vi "SWERVE DRIVE AUTO.vi"(8 "error in (no error)":errorcluster, 11 "auto pgm array":T4[](array[typedef])=[{"auto drive command"={"TRANSLATE"={"drive\ndistance (ft)"=10.0, "steer\nbearing (deg)"=0.0, "max strafe\nvelocity (ft/s)"=10.0, "max strafe\naccel (ft/s^2)"=58.7}, "ROTATE"={"rotate to\nbearing (deg)"=0.0, "max rotate\nvelocity (deg/s)"=0.0, "max rotate\naccel (ft/s^2)"=25.0}}, "sub-systems"={"start INTAKE"=FALSE, "extend FLAP"=FALSE, "SHOOT"=FALSE, "retract FLAP"=FALSE, "TARGET SPEAKER"=FALSE, "TARGET AMP"=FALSE, "TARGET OFF"=FALSE, "DANCE"=FALSE}}, {"auto drive command"={"TRANSLATE"={"drive\ndistance (ft)"=5.0, "steer\nbearing (deg)"=180.0, "max strafe\nvelocity (ft/s)"=5.0, "max strafe\naccel (ft/s^2)"=58.7}, "ROTATE"={"rotate to\nbearing (deg)"=0.0, "max rotate\nvelocity (deg/s)"=180.0, "max rotate\naccel (ft/s^2)"=25.0}}, "sub-systems"={"start INTAKE"=FALSE, "extend FLAP"=FALSE, "SHOOT"=FALSE, "retract FLAP"=FALSE, "TARGET SPEAKER"=FALSE, "TARGET AMP"=FALSE, "TARGET OFF"=FALSE, "DANCE"=FALSE}}] {"auto drive command"."ROTATE"."max rotate\naccel (ft/s^2)" min=0.0 max=200.0 step=0.1 format="%_3f"; "auto drive command"."ROTATE"."max rotate\nvelocity (deg/s)" min=0.0 step=0.001; "auto drive command"."TRANSLATE"."max strafe\naccel (ft/s^2)" min=0.0 max=200.0 step=0.1 format="%_3f"; "auto drive command"."TRANSLATE"."max strafe\nvelocity (ft/s)" min=0.0 max=20.0 step=0.001 format="%_5f"}) -> (0 "error out":errorcluster)   [LabVIEW 2023]
uses:
  ctrl defs/ctrl AUTONOMOUS step control.ctl
  ctrl defs/ctrl AUTONOMOUS drive step control.ctl
  ctrl defs/ctrl AUTONOMOUS systems step control.ctl
  ctrl defs/ctrl AUTO STATES.ctl
  <vilib>/Rock Robotics/WPI/ThirdParty/REV Robotics/REVLib/Typedef/Spark MAX Smart Motion Parameters.ctl
  <vilib>/Rock Robotics/WPI/ThirdParty/REV Robotics/REVLib/Typedef/Spark MAX Control Type.ctl
  Global INIT.vi
  Global odometry.vi
  <vilib>/Rock Robotics/WPI/ThirdParty/Phoenix-LabVIEW/CANCoder/Get/CTRE_Phoenix_CANcoder_GetSensorData.vi
  Global stack names.vi
  <vilib>/Rock Robotics/Network Tables/NT Read Boolean.vi
panel:
  out "Sensor Velocity":dbl[](array[numeric])
  in  "Smart Motion Parameters":T1
  in  "PID Constants":T2={"P Gain"=0.0, "I Gain"=0.0, "D Gain"=0.0, "F Gain"=0.0, "I Zone"=0.0, "Min Output"=-1.0, "Max Output"=1.0} {"Max Output" min=0.0 max=1.0 step=0.01; "Min Output" min=-1.0 max=0.0 step=0.01}
  in  "loop exit":bool
  in  "STATE":T3
  out "wheel\npos (rev)":dbl[](array[numeric])
  out "@ target":bool[](array[boolean])
  out "pos\ntarget (rev)":dbl[](array[numeric])
  out "rev tol\nto target":dbl
  out "distance (ft)\nto wheel revs":dbl
  out "vel to wheel\nspeed\n(rpm per ft/s)":dbl
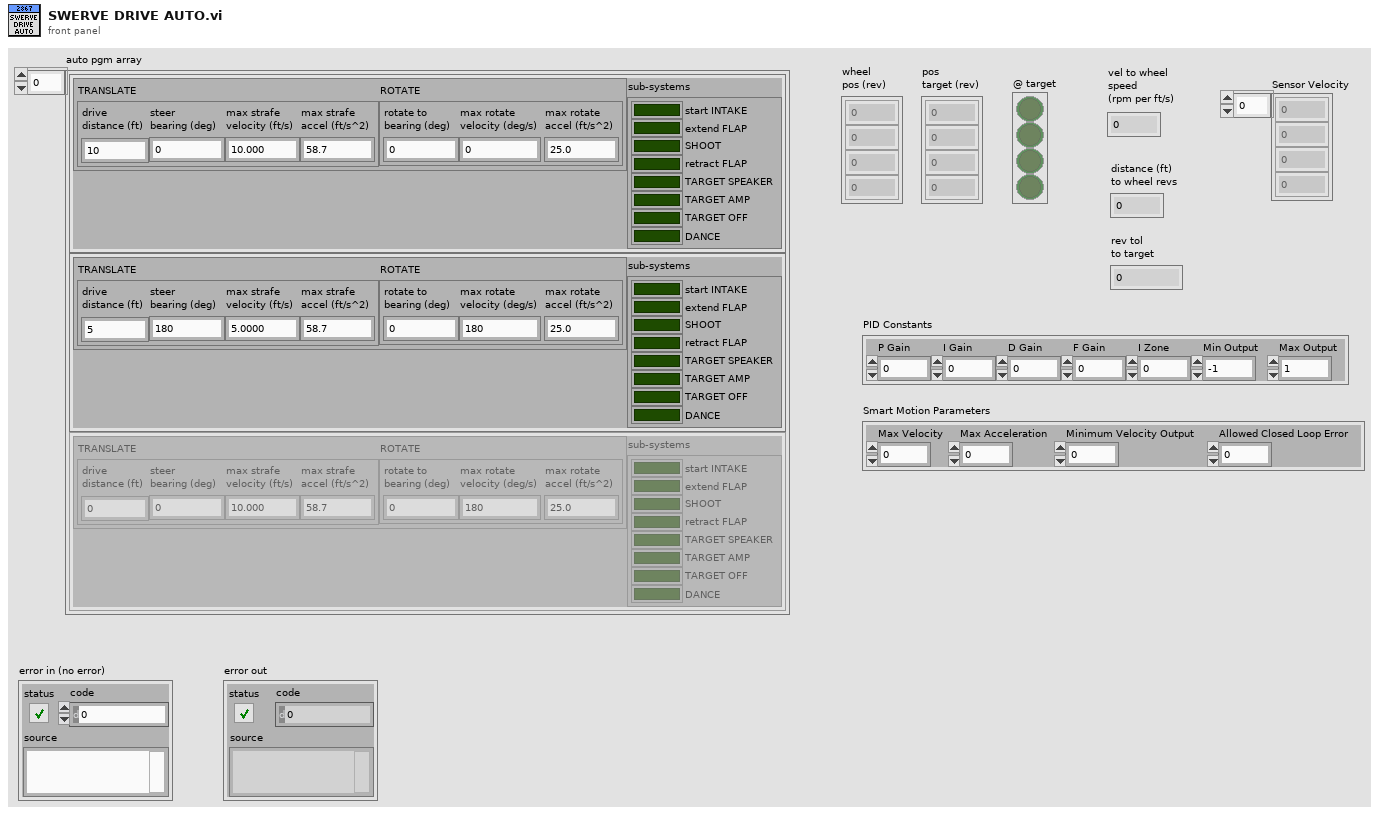
[diagram p1: front panel]
types:
  T1 = typedef "Spark MAX Smart Motion Parameters.ctl" = cluster{"Max Velocity":dbl, "Max Acceleration":dbl, "Minimum Velocity Output":dbl, "Allowed Closed Loop Error":dbl}
  T2 = cluster{"P Gain":dbl, "I Gain":dbl, "D Gain":dbl, "F Gain":dbl, "I Zone":dbl, "Min Output":dbl, "Max Output":dbl}
  T3 = typedef "ctrl AUTO STATES.ctl" = enum16{"TRANSLATE", "ROTATE", "TARGET", "INTAKE", "SHOOT", "DANCE", "WAIT for INTAKE", "WAIT for SHOOTER", "END", "SUB-SYSTEMS"}
  T4 = typedef "ctrl AUTONOMOUS step control.ctl" = cluster{"auto drive command":T5, "sub-systems":T6}
  T5 = typedef "ctrl AUTONOMOUS drive step control.ctl" = cluster{"TRANSLATE":cluster{"drive\ndistance (ft)":dbl, "steer\nbearing (deg)":dbl, "max strafe\nvelocity (ft/s)":dbl, "max strafe\naccel (ft/s^2)":dbl}, "ROTATE":cluster{"rotate to\nbearing (deg)":dbl, "max rotate\nvelocity (deg/s)":dbl, "max rotate\naccel (ft/s^2)":dbl}}
  T6 = typedef "ctrl AUTONOMOUS systems step control.ctl" = cluster{"start INTAKE":bool, "extend FLAP":bool, "SHOOT":bool, "retract FLAP":bool, "TARGET SPEAKER":bool, "TARGET AMP":bool, "TARGET OFF":bool, "DANCE":bool}
  T7 = typedef "ctrl swerve motor.ctl" = cluster{"description":string, "MOTOR SELECT":T8, "Installed?":bool, "CAN ID":u8, "refnum name":string, "Invert":bool, "Idle Mode":T9, "Current limiting":T10, "MOTOR PIDF coefficients":T11, "gear ratio":dbl}
  T8 = typedef "ctrl MOTOR SELECT.ctl" = i16
  T9 = typedef "Spark MAX Idle Mode.ctl" = enum16{"Coast", "Brake"}
  T10 = typedef "ctrl Spark MAX current limiting.ctl" = cluster{"Linearized":bool, "Free Speed (A)":dbl, "Primay (A)":dbl, "Limit RPM (0)":u32}
  T11 = typedef "ctrl motor PIDF coefficients.ctl" = cluster{"PIDF":cluster{"P Gain":dbl, "I Gain":dbl, "D Gain":dbl, "F Gain":dbl, "I Zone":dbl, "Min Output":dbl, "Max Output":dbl}, "Smart Motion":T1}
  T12 = typedef "ctrl swerve module.ctl" = cluster{"descr":string, "V":dbl, "POS":dbl, "target":dbl, "ABS":dbl, "from pivot to module":cluster{"R":dbl, "theta (deg)":dbl, "theta spin (deg)":dbl, "theta park (deg)":dbl}, "coord wrt geom CTR":cluster{"X":dbl, "Y":dbl}, "corner wt (lbm)":dbl}
  T13 = typedef "WPI_MotorControlDeviceRef.ctl" = cluster{"DeviceStatus":errorcluster, "Type":T14, "PWM":cluster{"PWM Channel":T15, "DeadBand":T16}, "CAN":cluster{"Device Number":u8, "SetOutput VI Ref":variant, "GetOutput VI Ref":variant, "Enable VI Ref":variant, "Disable VI Ref":variant, "Data":variant}, "Invert":bool, "DIO PWM":cluster{"PWM \"Enable\" Channel":T15, "DIOChannel":T17, "PWM Rate":dbl}}
  T14 = typedef "WPI_MotorControlType.ctl" = enum16{"PWM", "CAN", "DIO PWM"}
  T15 = typedef "FPGA_DIOPWMChannel.ctl" = enum8{"PWM 0", "PWM 1", "PWM 2", "PWM 3", "PWM 4", "PWM 5", "PWM 6", "PWM 7", "PWM 8", "PWM 9", "PWM MXP 0", "PWM MXP 1", "PWM MXP 2", "PWM MXP 3", "PWM MXP 4", "PWM MXP 5", "PWM MXP 6", "PWM MXP 7", "PWM MXP 8", "PWM MXP 9", "Invalid"}
  T16 = typedef "WPI_PWMDeadband.ctl" = cluster{"Name":string, "maxPositivePwm":i32, "minPositivePwm":i32, "centerPwm":i32, "maxNegativePwm":i32, "minNegativePwm":i32, "angularRange":u16}
  T17 = typedef "FPGA_DIOChannel.ctl" = enum8{"DIO 0", "DIO 1", "DIO 2", "DIO 3", "DIO 4", "DIO 5", "DIO 6", "DIO 7", "DIO 8", "DIO 9", "DIO MXP 0", "DIO MXP 1", "DIO MXP 2", "DIO MXP 3", "DIO MXP 4", "DIO MXP 5", "DIO MXP 6", "DIO MXP 7", "DIO MXP 8", "DIO MXP 9", "DIO MXP 10", "DIO MXP 11", "DIO MXP 12", "DIO MXP 13", "DIO MXP 14", "DIO MXP 15", "SPI Port CS1", "SPI Port CS2", "SPI Port CS3", "SPI Port MISO", "SPI Port MOSI", "Invalid"}
  T18 = typedef "CTRE_Phoenix_CANcoder_DeviceRef.ctl" = cluster{"DeviceStatus":errorcluster, "Device Number":u8, "Handle":u64, "UsageFrame":u32, "Library Path":path}
  T19 = cluster{"Driver":T13, "Steer":T13, "Encoder":T18}[]
  T20 = typedef "Spark MAX Control Type.ctl" = enum16{"Percent VBus", "Voltage", "Velocity", "Position", "Smart Motion", "Current", "Smart Velocity"}
  T21 = typedef "ctrl stack - INTAKE SHOOTER.ctl" = cluster{"INTAKE STATE":string, "RUN INTAKE?":string, "RUN REVERSE?":string, "NOTE LOADED?":string, "SHOOTER STATE":string, "SHOOTER FIRE?":string, "SHOOT AMP?":string, "EXTEND FLAP?":string, "LOOKING for NOTE":string}
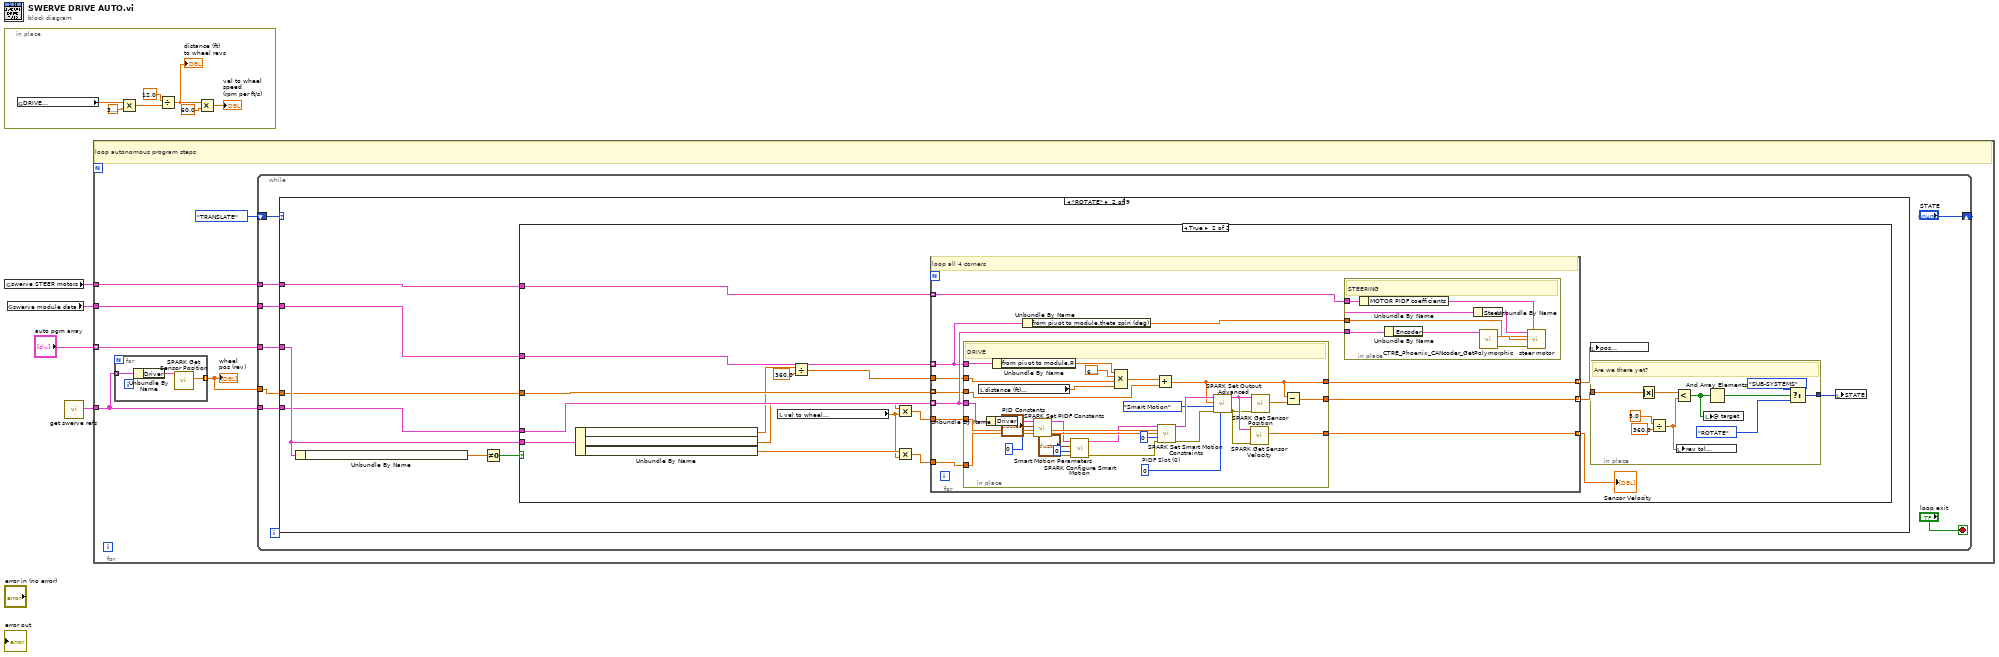
[diagram p0: block diagram]
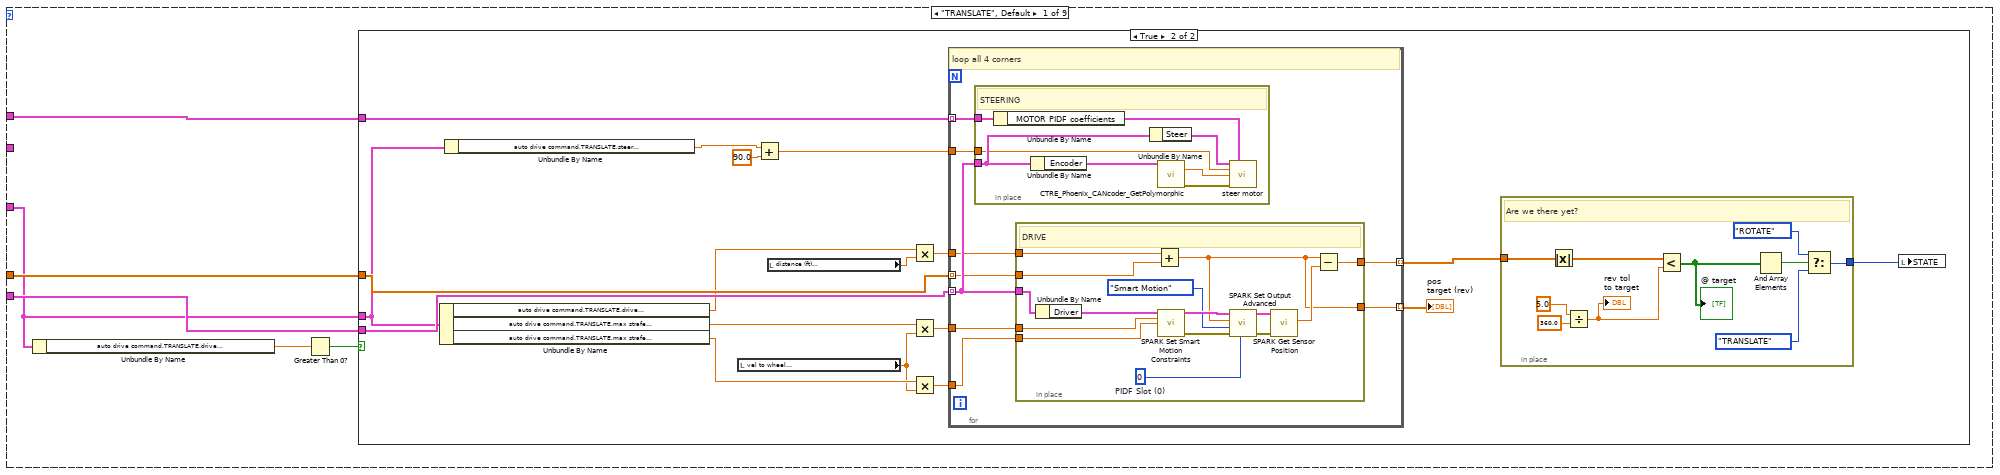
[diagram p2: hidden frame]
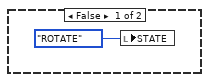
[diagram p3: hidden frame]
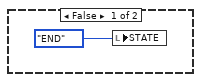
[diagram p4: hidden frame]
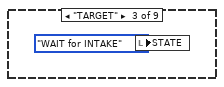
[diagram p5: hidden frame]
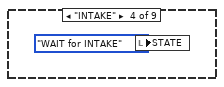
[diagram p6: hidden frame]
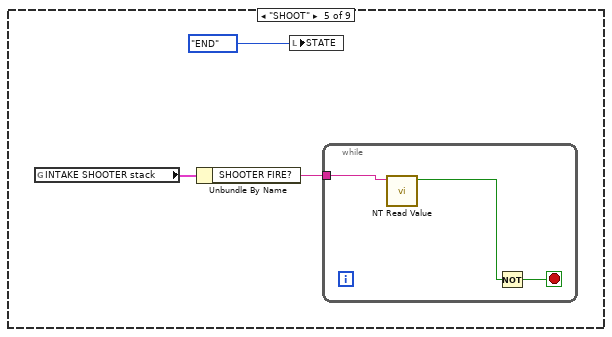
[diagram p7: hidden frame]
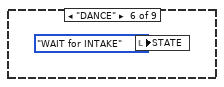
[diagram p8: hidden frame]
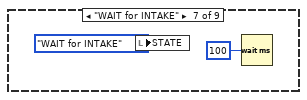
[diagram p9: hidden frame]
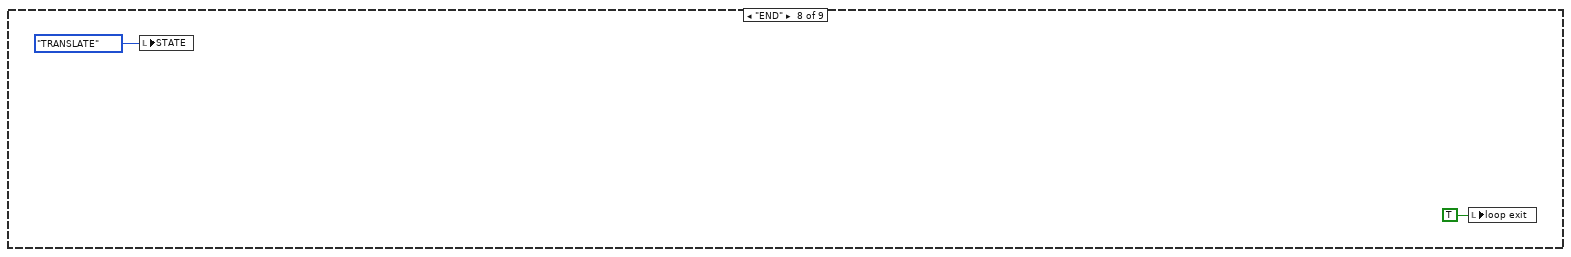
[diagram p10: hidden frame]
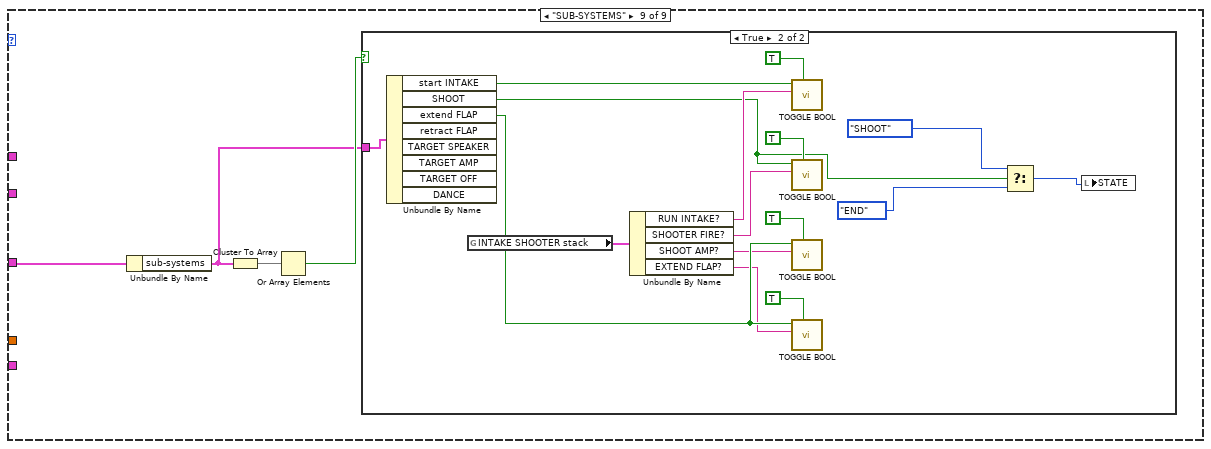
[diagram p11: hidden frame]
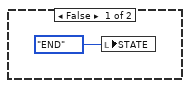
[diagram p12: hidden frame]
diagram:
  n1 = in-place {
    n2 = global read "Global INIT.vi" "DRIVE\nwheel diam (in)"() -> (w11:dbl)
    n3 = Multiply(x=w11, y=3.141592653589793) -> (x*y=w8:dbl)
    n4 = Divide(x=12.0, y=w8) -> (x/y=w7:dbl)
    "distance (ft)\nto wheel revs" <- w7
    n5 = Multiply(x=w7, y=60.0) -> (x*y=→"vel to wheel\nspeed\n(rpm per ft/s)":dbl)
  }
  n6 = global read "Global INIT.vi" "swerve STEER motors"() -> (w2:T7[])
  n7 = global read "Global odometry.vi" "swerve module data"() -> (w1:T12[])
  n8 = call "get swerve refs.vi"() -> ("Swerve refs"=w3:T19)  [unwired: 10 in, 1 out]
  n9 = for {
    tunnel: "auto pgm array" -> [w15] mode=indexing
    tunnel: w3 -> [w14]
    tunnel: w2 -> [w13]
    tunnel: w1 -> [w12]
    # "loop autonomous program steps"
    n10 = for {
      tunnel: w14 -> [w213] mode=indexing
      tunnel: [w211] -> w16 mode=indexing
      n11 = Unbundle By Name(w213) -> ("Driver"=w212:T13)
      n12 = call <vilib>:"SPARK Get Sensor Position.vi"("MotorControlDevRef in"=w212) -> ("Sensor Position"=w211:dbl)  [unwired: 7 in, 3 out]
    }
    "wheel\npos (rev)" <- w16
    n13 = while {
      shift-right: ["STATE"] -> _
      shift-left: ctrl_AUTO_STATES."TRANSLATE" -> [w25]
      tunnel: w16 -> [w22]
      tunnel: w15 -> [w24]
      tunnel: w14 -> [w23]
      tunnel: w13 -> [w21]
      tunnel: w12 -> [w20]
      stop <- "loop exit" stop-if-true
      n14 = case shown="\"ROTATE\"" w25 {
        tunnel: w24 -> [w26 w97 _ _ _ _ _ _ w193]
        tunnel: w23 -> [w29 w96 _ _ _ _ _ _ _]
        tunnel: w22 -> [w28 w95 _ _ _ _ _ _ _]
        tunnel: w21 -> [w27 w94 _ _ _ _ _ _ _]
        tunnel: w20 -> [_ w93 _ _ _ _ _ _ _]
        frame "TRANSLATE", Default {
          n15 = Unbundle By Name(w26) -> ("auto drive command.TRANSLATE.drive\ndistance (ft)"=w31:dbl)
          n16 = Greater Than 0?(x=w31) -> (x > 0?=w30:bool)
          n17 = case shown="True" w30 {
            tunnel: w29 -> [_ w50]
            tunnel: w28 -> [_ w49]
            tunnel: w27 -> [_ w48]
            tunnel: w26 -> [_ w47]
            frame False {
              n18 = local write "STATE"(ctrl_AUTO_STATES."ROTATE") -> ()
            }
            frame True {
              n19 = Unbundle By Name(w47) -> ("auto drive command.TRANSLATE.drive\ndistance (ft)"=w43:dbl, "auto drive command.TRANSLATE.max strafe\nvelocity (ft/s)"=w42:dbl, "auto drive command.TRANSLATE.max strafe\naccel (ft/s^2)"=w37:dbl)
              n20 = Unbundle By Name(w47) -> ("auto drive command.TRANSLATE.steer\nbearing (deg)"=w46:dbl)
              n21 = local read "vel to wheel\nspeed\n(rpm per ft/s)"() -> (w36:dbl)
              n22 = Add(x=w46, y=90.0) -> (x+y=w44:dbl)
              n23 = local read "distance (ft)\nto wheel revs"() -> (w41:dbl)
              n24 = Multiply(x=w43, y=w41) -> (x*y=w40:dbl)
              n25 = Multiply(x=w42, y=w36) -> (x*y=w39:dbl)
              n26 = Multiply(x=w37, y=w36) -> (x*y=w38:dbl)
              n27 = for {
                tunnel: w50 -> [w67] mode=indexing
                tunnel: w49 -> [w63] mode=indexing
                tunnel: w48 -> [w68] mode=indexing
                tunnel: w44 -> [w69]
                tunnel: w40 -> [w66]
                tunnel: w39 -> [w64]
                tunnel: w38 -> [w65]
                tunnel: [w62] -> w35 mode=indexing
                tunnel: [w61] -> w34 mode=indexing
                # "loop all 4 corners"
                n28 = in-place {
                  in-place-border: w67 -> [w89]
                  in-place-border: w69 -> [w88]
                  in-place-border: w68 -> [w86]
                  # "STEERING"
                  n29 = Unbundle By Name(w86) -> ("MOTOR PIDF coefficients"=w85:T11)
                  n30 = Unbundle By Name(w89) -> ("Encoder"=w92:T18)
                  n31 = Unbundle By Name(w89) -> ("Steer"=w90:T13)
                  n32 = call-poly <vilib>:"CTRE_Phoenix_CANcoder_GetPolymorphic.vi"("CTRE_CANcoder_DeviceRef"=w92) -> ("Position"=w91:dbl, "error out"=w87:errorcluster)  [unwired: 10 in, 3 out]
                  n33 = call "steer motor.vi"("MotorControlDevRef"=w90, "MOTOR PIDF coefficients"=w85, "target"=w88, "encoder"=w91, "error in (no error)"=w87) -> ()  [unwired: 10 in, 1 out]
                }
                n34 = in-place {
                  in-place-border: w67 -> [w80]
                  in-place-border: w66 -> [w78]
                  in-place-border: w65 -> [w76]
                  in-place-border: w64 -> [w77]
                  in-place-border: w63 -> [w75]
                  in-place-border: [w71] -> w62
                  in-place-border: [w70] -> w61
                  w81 = 0  # PIDF Slot (0)
                  # "DRIVE"
                  n35 = Unbundle By Name(w80) -> ("Driver"=w79:T13)
                  n36 = Add(x=w78, y=w75) -> (x+y=w70:dbl)
                  n37 = call <vilib>:"SPARK Set Smart Motion Constraints.vi"("MotorControlDeviceRef"=w79, "Max Velocity"=w77, "Max Acceleration"=w76) -> ("MotorControlDeviceRef"=w83:T13, "error out"=w84:errorcluster)  [unwired: 11 in]
                  n38 = call <vilib>:"SPARK Set Output Advanced.vi"("PIDF Slot (0)"=w81, "error in (no error)"=w84, "Control Mode"=Spark_MAX_Control_Type."Smart Motion", "Setpoint"=w70, "MotorControlDevRef"=w83) -> ("error out"=w74:errorcluster, "MotorControlDevRef"=w73:T13)  [unwired: 5 in]
                  n39 = call <vilib>:"SPARK Get Sensor Position.vi"("error in (no error)"=w74, "MotorControlDevRef in"=w73) -> ("Sensor Position"=w72:dbl)  [unwired: 6 in, 3 out]
                  n40 = Subtract(x=w70, y=w72) -> (x-y=w71:dbl)
                }
              }
              "pos\ntarget (rev)" <- w34
              n41 = in-place {
                in-place-border: w35 -> [w60]
                in-place-border: [w56] -> w33
                # "Are we there yet?"
                n42 = Absolute Value(x=w60) -> (abs(x)=w55:dbl[])
                n43 = Divide(x=5.0, y=360.0) -> (x/y=w54:dbl)
                "rev tol\nto target" <- w54
                n44 = Less?(x=w55, y=w54) -> (x < y?=w51:bool[])
                "@ target" <- w51
                n45 = And Array Elements(Boolean array=w51) -> (logical AND=w59:bool)
                n46 = Select(t=ctrl_AUTO_STATES."ROTATE", s=w59, f=ctrl_AUTO_STATES."TRANSLATE") -> (s? t:f=w56:T3)
              }
              n47 = local write "STATE"(w33) -> ()
            }
          }
        }
        frame "ROTATE" {
          n48 = Unbundle By Name(w97) -> ("auto drive command.ROTATE.rotate to\nbearing (deg)"=w99:dbl)
          n49 = Not Equal To 0?(x=w99) -> (x != 0?=w98:bool)
          n50 = case shown="True" w98 {
            tunnel: w96 -> [_ w117]
            tunnel: w95 -> [_ w116]
            tunnel: w94 -> [_ w115]
            tunnel: w97 -> [_ w114]
            tunnel: w93 -> [_ w107]
            frame False {
              n51 = local write "STATE"(ctrl_AUTO_STATES."END") -> ()
            }
            frame True {
              n52 = Unbundle By Name(w114) -> ("auto drive command.ROTATE.rotate to\nbearing (deg)"=w106:dbl, "auto drive command.ROTATE.max rotate\nvelocity (deg/s)"=w113:dbl, "auto drive command.ROTATE.max rotate\naccel (ft/s^2)"=w110:dbl)
              n53 = local read "vel to wheel\nspeed\n(rpm per ft/s)"() -> (w109:dbl)
              n54 = Divide(x=w106, y=360.0) -> (x/y=w104:dbl)
              n55 = Multiply(x=w113, y=w109) -> (x*y=w112:dbl)
              n56 = Multiply(x=w110, y=w109) -> (x*y=w111:dbl)
              n57 = for {
                tunnel: w117 -> [w137] mode=indexing
                tunnel: w116 -> [w134] mode=indexing
                tunnel: w115 -> [w138] mode=indexing
                tunnel: w112 -> [w135]
                tunnel: w111 -> [w136]
                tunnel: [w133] -> w108 mode=indexing
                tunnel: [w132] -> w103 mode=indexing
                tunnel: w107 -> [w130] mode=indexing
                tunnel: w104 -> [w129]
                tunnel: [w128] -> w101 mode=indexing
                # "loop all 4 corners"
                n58 = in-place {
                  in-place-border: w137 -> [w164]
                  in-place-border: w136 -> [w161]
                  in-place-border: w135 -> [w162]
                  in-place-border: w134 -> [w160]
                  in-place-border: [w158] -> w133
                  in-place-border: [w157] -> w132
                  in-place-border: w130 -> [w156]
                  in-place-border: w129 -> [w153]
                  in-place-border: [w139] -> w128
                  w165 = 0  # PIDF Slot (0)
                  # "DRIVE"
                  n59 = local read "distance (ft)\nto wheel revs"() -> (w152:dbl)
                  n60 = Unbundle By Name(w164) -> ("Driver"=w163:T13)
                  n61 = Unbundle By Name(w156) -> ("from pivot to module.R"=w155:dbl)
                  n62 = call <vilib>:"SPARK Set PIDF Constants.vi"("PIDF Slot"=0, "PID Constants"="PID Constants", "MotorControlDeviceRef"=w163) -> ("error out"=w146:errorcluster, "MotorControlDeviceRef"=w148:T13)  [unwired: 7 in]
                  n63 = call <vilib>:"SPARK Configure Smart Motion.vi"("error in"=w146, "PIDF Slot (0)"=0, "Smart Motion Parameters"="Smart Motion Parameters", "MotorControlDeviceRef"=w148) -> ("error out"=w145:errorcluster, "MotorControlDeviceRef"=w147:T13)  [unwired: 6 in]
                  n64 = Compound Arithmetic op=MULTIPLY(w155, 6.283185307179586, w153, w152) -> (w151:dbl)
                  n65 = Add(x=w151, y=w160) -> (x+y=w157:dbl)
                  n66 = call <vilib>:"SPARK Set Smart Motion Constraints.vi"("MotorControlDeviceRef"=w147, "Max Velocity"=w162, "Max Acceleration"=w161, "PIDF Slot (0)"=0, "error in"=w145) -> ("MotorControlDeviceRef"=w167:T13, "error out"=w168:errorcluster)  [unwired: 9 in]
                  n67 = call <vilib>:"SPARK Set Output Advanced.vi"("PIDF Slot (0)"=w165, "error in (no error)"=w168, "Control Mode"=Spark_MAX_Control_Type."Smart Motion", "Setpoint"=w157, "MotorControlDevRef"=w167) -> ("error out"=w140:errorcluster, "MotorControlDevRef"=w141:T13)  [unwired: 5 in]
                  n68 = call <vilib>:"SPARK Get Sensor Velocity.vi"("error in (no error)"=w140, "MotorControlDevRef in"=w141) -> ("Sensor Velocity"=w139:dbl)  [unwired: 6 in, 3 out]
                  n69 = call <vilib>:"SPARK Get Sensor Position.vi"("error in (no error)"=w140, "MotorControlDevRef in"=w141) -> ("Sensor Position"=w159:dbl)  [unwired: 6 in, 3 out]
                  n70 = Subtract(x=w157, y=w159) -> (x-y=w158:dbl)
                }
                n71 = Unbundle By Name(w130) -> ("from pivot to module.theta spin (deg)"=w131:dbl)
                n72 = in-place {
                  in-place-border: w137 -> [w173]
                  in-place-border: w138 -> [w171]
                  in-place-border: w131 -> [w169]
                  # "STEERING"
                  n73 = Unbundle By Name(w171) -> ("MOTOR PIDF coefficients"=w170:T11)
                  n74 = Unbundle By Name(w173) -> ("Encoder"=w176:T18)
                  n75 = Unbundle By Name(w173) -> ("Steer"=w174:T13)
                  n76 = call-poly <vilib>:"CTRE_Phoenix_CANcoder_GetPolymorphic.vi"("CTRE_CANcoder_DeviceRef"=w176) -> ("Position"=w175:dbl, "error out"=w172:errorcluster)  [unwired: 10 in, 3 out]
                  n77 = call "steer motor.vi"("MotorControlDevRef"=w174, "MOTOR PIDF coefficients"=w170, "target"=w169, "encoder"=w175, "error in (no error)"=w172) -> ()  [unwired: 10 in, 1 out]
                }
              }
              "Sensor Velocity" <- w101
              n78 = local write "pos\ntarget (rev)"(w103) -> ()
              n79 = in-place {
                in-place-border: w108 -> [w127]
                in-place-border: [w123] -> w102
                # "Are we there yet?"
                n80 = Absolute Value(x=w127) -> (abs(x)=w122:dbl[])
                n81 = Divide(x=5.0, y=360.0) -> (x/y=w119:dbl)
                n82 = Less?(x=w122, y=w119) -> (x < y?=w118:bool[])
                n83 = local write "rev tol\nto target"(w119) -> ()
                n84 = local write "@ target"(w118) -> ()
                n85 = And Array Elements(Boolean array=w118) -> (logical AND=w126:bool)
                n86 = Select(t=ctrl_AUTO_STATES."SUB-SYSTEMS", s=w126, f=ctrl_AUTO_STATES."ROTATE") -> (s? t:f=w123:T3)
              }
              n87 = local write "STATE"(w102) -> ()
            }
          }
        }
        frame "TARGET" {
          n88 = local write "STATE"(ctrl_AUTO_STATES."WAIT for INTAKE") -> ()
        }
        frame "INTAKE" {
          n89 = local write "STATE"(ctrl_AUTO_STATES."WAIT for INTAKE") -> ()
        }
        frame "SHOOT" {
          n90 = global read "Global stack names.vi" "INTAKE SHOOTER stack"() -> (w180:T21)
          n91 = Unbundle By Name(w180) -> ("SHOOTER FIRE?"=w179:string)
          n92 = local write "STATE"(ctrl_AUTO_STATES."END") -> ()
          n93 = while {
            tunnel: w179 -> [w184]
            stop <- w182 stop-if-true
            n94 = call-poly <vilib>:"NT Read Value.vi"("name"=w184) -> ("value"=w183:bool)  [unwired: 8 in, 2 out]
            n95 = Not(x=w183) -> (.not. x?=w182:bool)
          }
        }
        frame "DANCE" {
          n96 = local write "STATE"(ctrl_AUTO_STATES."WAIT for INTAKE") -> ()
        }
        frame "WAIT for INTAKE" {
          n97 = local write "STATE"(ctrl_AUTO_STATES."WAIT for INTAKE") -> ()
          n98 = Wait (ms)(milliseconds to wait=u32 100) -> ()  [unwired: 1 out]
        }
        frame "END" {
          n99 = local write "STATE"(ctrl_AUTO_STATES."TRANSLATE") -> ()
          n100 = local write "loop exit"(TRUE) -> ()
        }
        frame "SUB-SYSTEMS" {
          n101 = Unbundle By Name(w193) -> ("sub-systems"=w190:T6)
          n102 = Cluster To Array(cluster=w190) -> (array=w192:bool[])
          n103 = Or Array Elements(Boolean array=w192) -> (logical OR=w191:bool)
          n104 = case shown="True" w191 {
            tunnel: w190 -> [_ w210]
            frame False {
              n105 = local write "STATE"(ctrl_AUTO_STATES."END") -> ()
            }
            frame True {
              n106 = Unbundle By Name(w210) -> ("start INTAKE"=w208:bool, "SHOOT"=w198:bool, "extend FLAP"=w209:bool)  [unwired: 5 out]
              n107 = global read "Global stack names.vi" "INTAKE SHOOTER stack"() -> (w207:T21)
              n108 = Unbundle By Name(w207) -> ("RUN INTAKE?"=w204:string, "SHOOTER FIRE?"=w205:string, "SHOOT AMP?"=w206:string, "EXTEND FLAP?"=w203:string)
              n109 = call "TOGGLE BOOL.vi"("force"=TRUE, "stack ref name"=w204, "Button Pressed?"=w208) -> ()  [unwired: 8 in, 1 out]
              n110 = call "TOGGLE BOOL.vi"("force"=TRUE, "stack ref name"=w205, "Button Pressed?"=w198) -> ()  [unwired: 8 in, 1 out]
              n111 = call "TOGGLE BOOL.vi"("force"=TRUE, "stack ref name"=w206, "Button Pressed?"=w209) -> ()  [unwired: 8 in, 1 out]
              n112 = call "TOGGLE BOOL.vi"("force"=TRUE, "stack ref name"=w203, "Button Pressed?"=w209) -> ()  [unwired: 8 in, 1 out]
              n113 = Select(t=ctrl_AUTO_STATES."SHOOT", s=w198, f=ctrl_AUTO_STATES."END") -> (s? t:f=w195:T3)
              n114 = local write "STATE"(w195) -> ()
            }
          }
        }
      }
    }
  }
